vi "Close_Spectrometer.vi"(1 "Spectr* In":u32, 2 "error in (no error)":errorcluster) -> (0 "error out":errorcluster)   [LabVIEW 2012]
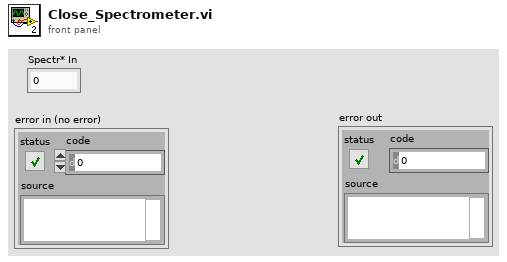
[diagram p1: front panel]
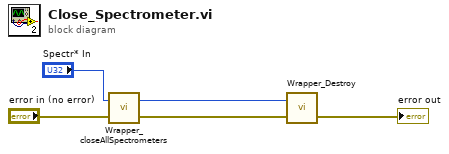
[diagram p0: block diagram]
diagram:
  n1 = call "Wrapper_closeAllSpectrometers.vi"("error in (no error)"="error in (no error)", "Wrapper In"="Spectr* In") -> ("error out"=w3:errorcluster, "Wrapper Out"=w5:u32)
  n2 = call "Wrapper_Destroy.vi"("error in (no error)"=w3, "Wrapper"=w5) -> ("error out"=→"error out":errorcluster)  [unwired: 1 in]
